vi "Double_click.vi"(8 "error in":errorcluster) -> (0 "error out":errorcluster)   [LabVIEW 2024]
panel:
  in  "OK, got it!":bool
  # "Double click!"
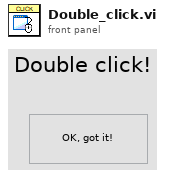
[diagram p1: front panel]
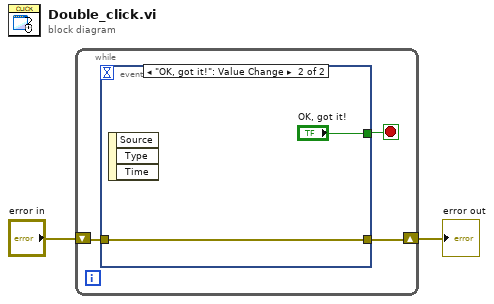
[diagram p0: block diagram]
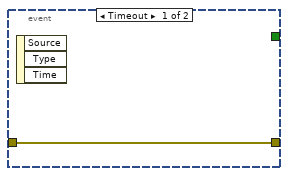
[diagram p2: hidden frame]
diagram:
  n1 = while {
    shift-right: [w4] -> w2
    shift-left: "error in" -> [w3]
    stop <- w5 stop-if-true
    n2 = event shown="[1] \"OK, got it!\": Value Change" {
      selector: _ -> [_ _]
      dyn-events: _ -> [_ _]
      timeout: _ -> [_ _]
      tunnel: [_ "OK, got it!"] -> w5
      tunnel: [w6 w7] -> w4
      tunnel: w3 -> [w6 w7]
      event Timeout {
        n3 = event-data() -> ()  [unwired: 1 in, 3 out]
      }
      event "OK, got it!": Value Change {
        n4 = event-data() -> ()  [unwired: 1 in, 3 out]
      }
    }
  }
  "error out" <- w2
